vi "Reset Timer.vi"(8 "error in (no error)":errorcluster, 11 "Timer Demo App in":refnum<class "Timer Demo App.lvclass">) -> (0 "error out":errorcluster, 3 "Timer Demo App out":refnum<class "Timer Demo App.lvclass">)   [LabVIEW 2020, in "Timer Demo.lvlib" / "Timer Demo App.lvclass"]
uses:
  Timer Demo App.lvclass
  Timer Demo App.lvclass/Timer Demo App.ctl
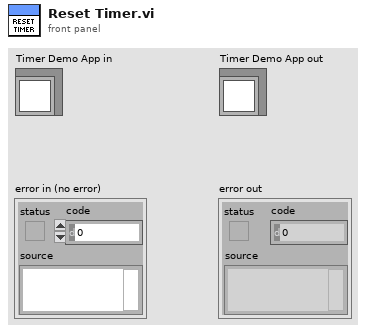
[diagram p1: front panel]
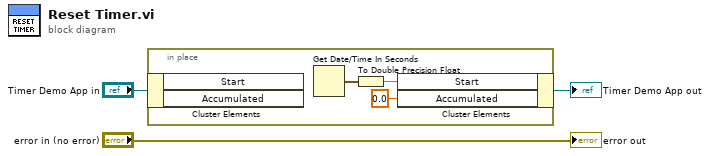
[diagram p0: block diagram]
diagram:
  n1 = in-place {
    n2 = in-place-cluster #1("Timer Demo App in") -> ()  [unwired: 2 out]
    n3 = Get Date/Time In Seconds() -> (seconds since 1Jan1904=w5:timestamp)
    n4 = To Double Precision Float(number=w5) -> (double precision float=w4:dbl)
    n5 = in-place-cluster #1("Start"=w4, "Accumulated"=0.0 ("Timer State.Accumulated")) -> (→"Timer Demo App out":refnum<class "Timer Demo App.lvclass">)
  }
  "error out" <- "error in (no error)"
